vi "from string.vi"(8 "error in":errorcluster, 9 "data":string, 10 "version":string, 11 "user tag bus module configuration In":refnum<class "fixed channel tag bus module configuration.lvclass">) -> (0 "error out":errorcluster, 3 "user tag bus module configuration Out":refnum<class "fixed channel tag bus module configuration.lvclass">)   [LabVIEW 2013]
doc: "Provides an interface for loading a module configuration from a file or other serialized data source. It is recommended that all children of this class store data in two sets--data required for its own initialization, and any data required for parent initialization--and that each implementation uses the <b>Call Parent Method</b> primitive to de-serialize parent information. As a result, it is expected that every module configuration class calls <b>component configuration.lvclass:From String.vi</b>."
uses:
  <vilib>/NI/Tag Bus Module Framework/root configuration/TBM configuration.lvclass
  <vilib>/NI/Tag Bus Module Framework/module configuration/TBM module configuration.lvclass
  fixed channel tag bus module configuration.lvclass
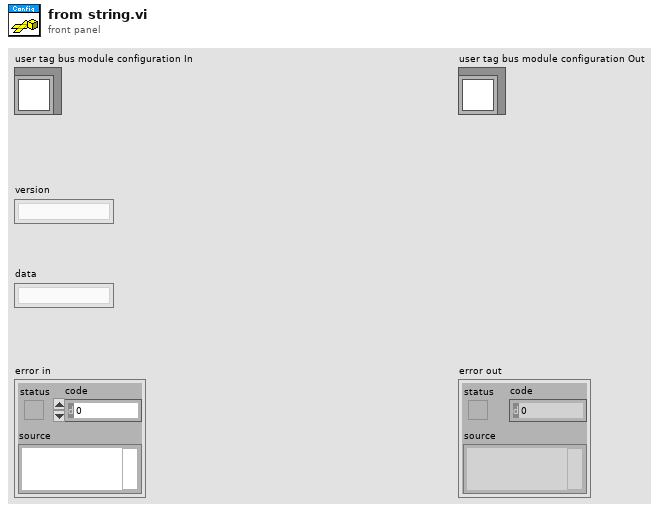
[diagram p1: front panel]
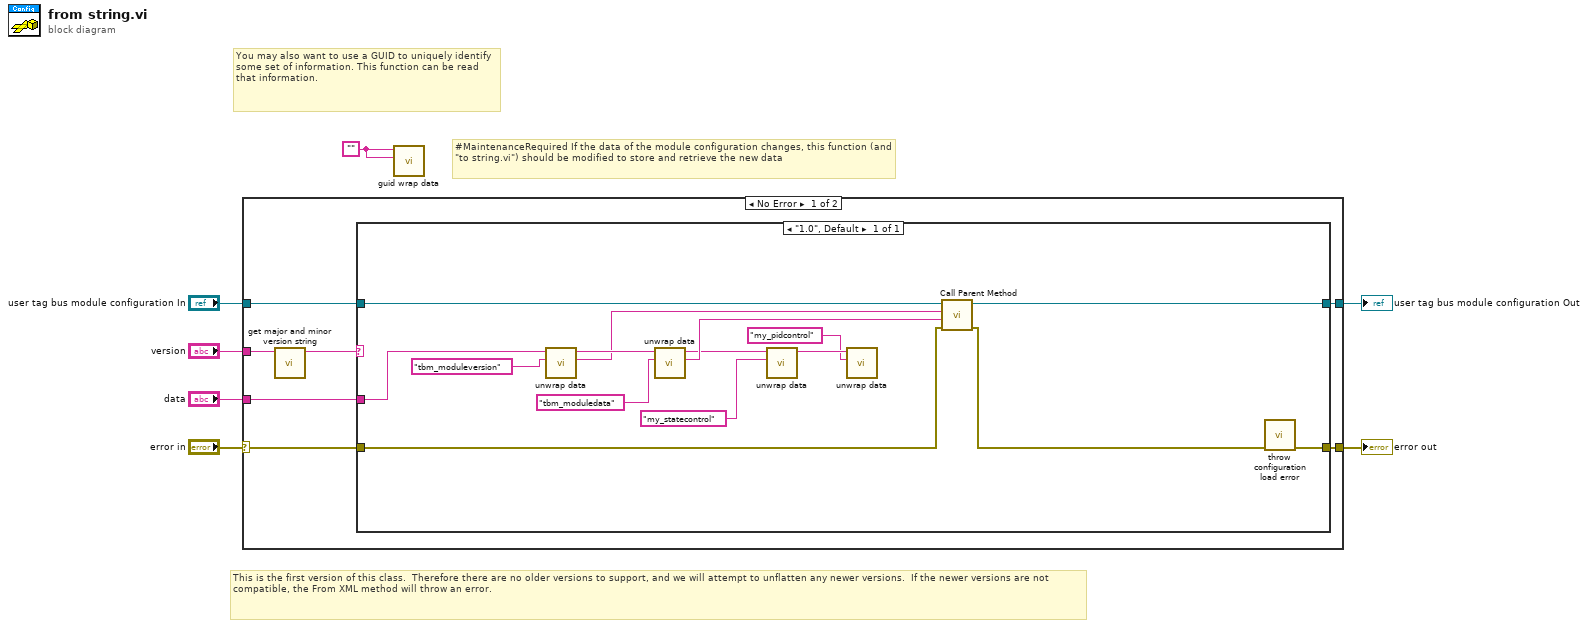
[diagram p0: block diagram]
diagram:
  w1 = ""
  # "You may also want to use a GUID to uniquely identify some set of information. This function can be read that information."
  # "#MaintenanceRequired If the data of the module configuration changes, this function (and \"to string.vi\") should be modified to store and retrieve the new data"
  # "This is the first version of this class.  Therefore there are no older versions to support, and we will attempt to unflatten any newer versions.  If the newer versions are not compatible, the From XML method will throw an error."
  n1 = case shown="No Error" "error in" {
    selector: "error in" -> [w8 w33]
    tunnel: "data" -> [w14 _]
    tunnel: "user tag bus module configuration In" -> [w13 w32]
    tunnel: [w12 w32] -> w6
    tunnel: [w11 w33] -> w5
    tunnel: "version" -> [w10 _]
    frame No Error {
      n2 = call <vilib>:"get major and minor version string.vi"("full version"=w10) -> ("major.minor version"=w9:string)  [unwired: 10 in]
      n3 = case shown="\"1.0\", Default" w9 {
        tunnel: w14 -> [w28]
        tunnel: w8 -> [w27]
        tunnel: w13 -> [w31]
        tunnel: [w16] -> w12
        tunnel: [w30] -> w11
        frame "1.0", Default {
          n4 = call <vilib>:"unwrap data.vi"("identifier"="tbm_moduleversion" ("additional identifier"), "data to unwrap"=w28) -> ("unwrapped data"=w23:string, "remaining string"=w29:string)  [unwired: 8 in]
          n5 = call <vilib>:"unwrap data.vi"("identifier"="tbm_moduledata" ("additional identifier"), "data to unwrap"=w29) -> ("unwrapped data"=w25:string, "remaining string"=w22:string)  [unwired: 8 in]
          n6 = call <vilib>:"unwrap data.vi"("identifier"="my_statecontrol" ("additional identifier"), "data to unwrap"=w22) -> ("unwrapped data"=w20:string, "remaining string"=w19:string)  [unwired: 8 in]
          n7 = call <vilib>:"unwrap data.vi"("identifier"="my_pidcontrol" ("additional identifier"), "data to unwrap"=w19) -> ("unwrapped data"=w17:string)  [unwired: 8 in, 1 out]
          n8 = call-parent "Call Parent Method"("error in"=w27, "data"=w25, "version"=w23, "module configuration in"=w31) -> ("error out"=w15:errorcluster, "module configuration out"=w16:refnum<class "fixed channel tag bus module configuration.lvclass">)  [unwired: 6 in]
          n9 = call <vilib>:"throw configuration load error.vi"("error in"=w15) -> ("error out"=w30:errorcluster)  [unwired: 10 in]
        }
      }
    }
    frame Error {
    }
  }
  "error out" <- w5
  "user tag bus module configuration Out" <- w6
  n10 = call <vilib>:"guid wrap data.vi"("identifier"=w1, "data to wrap"=w1) -> ()  [unwired: 8 in, 2 out]
